vi "Queue Receive.vi"(11 "Base Queue Actor in":refnum<class "Base Queue Actor.lvclass">) -> (2 "Msg":refnum<class "Msg.lvclass">, 3 "Base Queue Actor out":refnum<class "Base Queue Actor.lvclass">)   [LabVIEW 2021, in "jettl.lvlib" / "Base Queue Actor.lvclass"]
uses:
  Base Queue Actor.lvclass
  Msg/Msg/Msg.lvclass
  Base Queue Actor.lvclass/Base Queue Actor.ctl
  jettl.lvlib
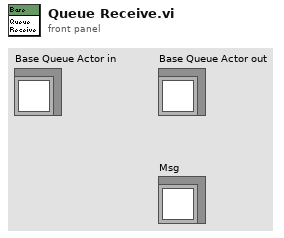
[diagram p1: front panel]
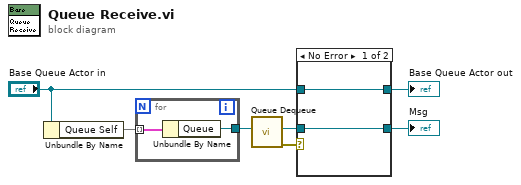
[diagram p0: block diagram]
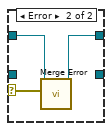
[diagram p2: hidden frame]
diagram:
  n1 = Unbundle By Name("Base Queue Actor in") -> ("Queue Self"=w2:map{string, refnum<data-value>})
  n2 = for {
    tunnel: w2 -> [w9] mode=indexing
    tunnel: [w8] -> w1
    n3 = Unbundle By Name(w9) -> ("Queue"=w8:refnum<data-value>)
  }
  n4 = call "Queue Dequeue.vi"("Queue"=w1) -> ("error out"=w7:errorcluster, "Msg"=w6:refnum<class "Msg.lvclass">)  [unwired: 9 in]
  n5 = case shown="No Error" w7 {
    selector: w7 -> [_ w12]
    tunnel: w6 -> [w10 _]
    tunnel: "Base Queue Actor in" -> [w11 w14]
    tunnel: [w11 w13] -> w5
    tunnel: [w10 _] -> w4
    frame No Error {
    }
    frame Error {
      n6 = call-dynamic "Merge Error.vi"("Error"=w12, "Base Queue Actor in"=w14) -> ("Base Queue Actor out"=w13:refnum<class "Base Queue Actor.lvclass">)  [unwired: 9 in]
    }
  }
  "Base Queue Actor out" <- w5
  "Msg" <- w4
